vi "DDsDefaltPath.vi"(8 "error in (no error)":errorcluster) -> (0 "error out":errorcluster, 3 "Default path":path)   [LabVIEW 2020, in "Other.lvlib"]
uses:
  Other.lvlib
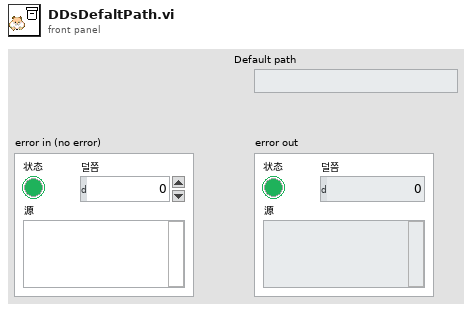
[diagram p1: front panel]
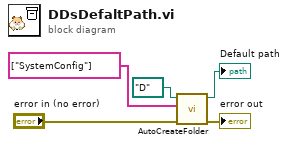
[diagram p0: block diagram]
diagram:
  n1 = call "AutoCreateFolder.vi"("error in (no error)"="error in (no error)", "Names"=string[] ["SystemConfig"], "Base path"=path "D:/") -> ("error out"=→"error out":errorcluster, "Created path"=→"Default path":path)  [unwired: 7 in]
